vi "Tx_Create FIFO Association - Cyclic Labels - Disable Channels.vi"(8 "error in (no error)":errorcluster, 11 "Input Channel Data []":T3[](array[typedef]) {"Labels Settings"."Label Timestamp Channel Data Reference" format="%.0x"; "Labels Settings"."Label Disable/Trigger Channel Reference" format="%.0x"; "Labels Settings"."Word"."Param Setting"."Item Refs" format="%.0x"; "Labels Settings"."Word"."Param Setting"."Num Bits" min=1 max=32; "Labels Settings"."Word"."Param Setting"."Start Bit" min=8 max=31; "Labels Settings"."Label" format="%.0o"}) -> (0 "error out":errorcluster, 3 "Cyclic Labels - Disable Channels Map":T1[](array[typedef]) {"Channel Data Reference" format="%.0x"})   [LabVIEW 2016, in "Ballard Arinc-429 Engine.lvlib"]
doc: "This VI creates a static association between NI-VS FIFO Channel Index and Physical Channel, Label Index, of disable channel for a Tx Scheduled Label."
uses:
  Ballard Arinc-429 Engine.lvlib
  Shared/Controls and Global/RT HW Channel.ctl
  Shared/Controls and Global/RT Label Settings.ctl
  Shared/Controls and Global/Label.ctl
  Shared/Controls and Global/transferPeriod.ctl
  Shared/Controls and Global/RT Word Settings.ctl
  Shared/Controls and Global/RT Param Setting.ctl
  Shared/Controls and Global/Start Bit.ctl
  Shared/Controls and Global/Number of Bits.ctl
  <vilib>/NI Veristand/Custom Device API/Block Data Reference.ctl
  <vilib>/NI Veristand/Custom Device API/Data Reference.ctl
  <vilib>/NI Veristand/Custom Device API/Custom Device Item Ref.ctl
  Shared/Controls and Global/TransferType.ctl
  RT Controls/RT Tx Association.ctl
  <vilib>/NI VeriStand/Custom Device API/Custom Device API.lvlib
  Shared/Ballard Arinc-429 Shared.lvlib
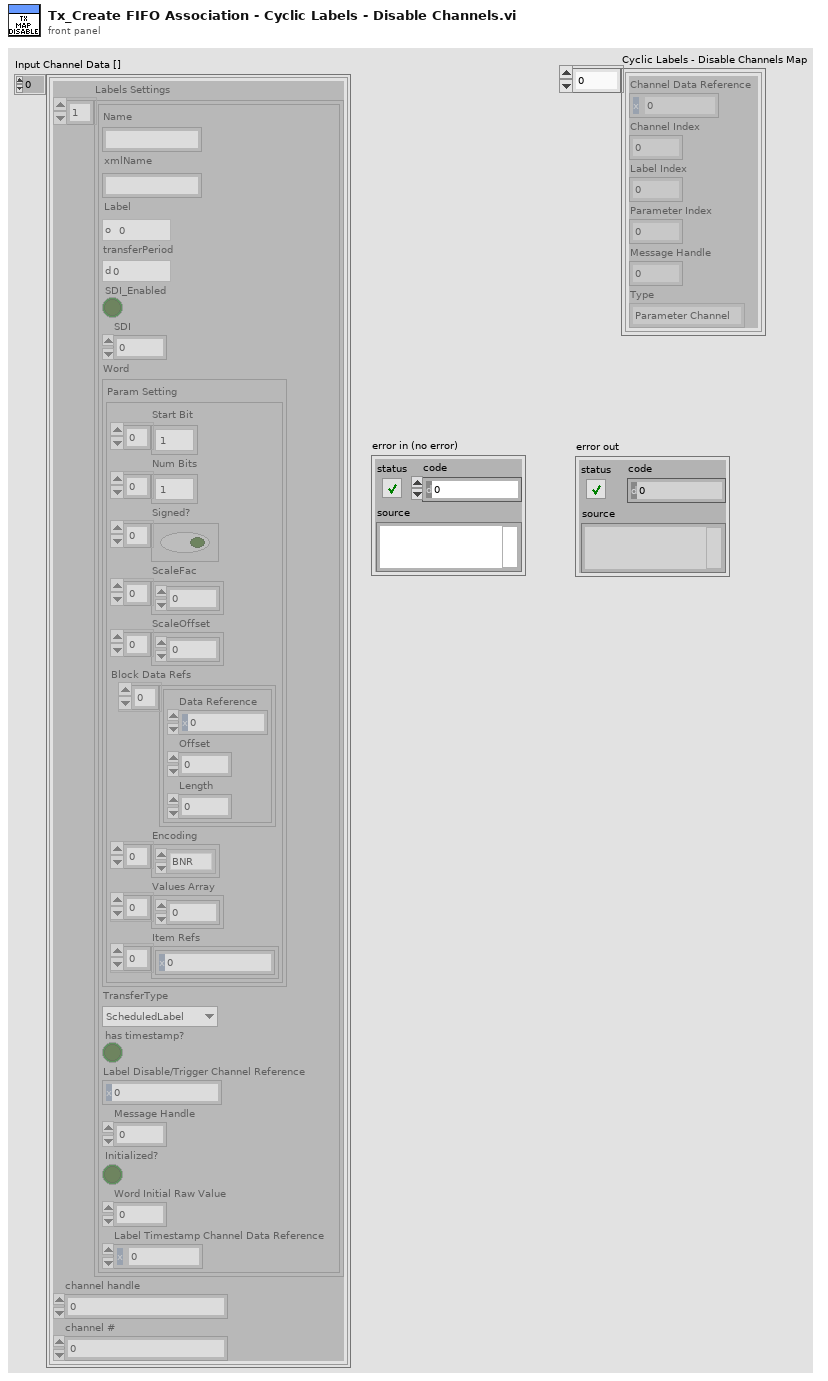
[diagram p1: front panel]
types:
  T1 = typedef "Ballard Arinc-429 Engine.lvlib/RT Tx Association.ctl" = cluster{"Channel Data Reference":T2, "Channel Index":i32, "Label Index":i32, "Parameter Index":i32, "Message Handle":u64, "Type":enum16{"Parameter Channel", "Disable/Trigger Channel"}}
  T2 = typedef "Custom Device API.lvlib/Data Reference.ctl" = i32
  T3 = typedef "Ballard Arinc-429 Shared.lvlib/RT HW Channel.ctl" = cluster{"Labels Settings":T4[], "channel handle":u64, "channel #":u16}
  T4 = typedef "Ballard Arinc-429 Shared.lvlib/RT Label Settings.ctl" = cluster{"Name":string, "xmlName":string, "Label":T5, "transferPeriod":T6, "SDI_Enabled":bool, "SDI":u8, "Word":T7, "TransferType":T13, "has timestamp?":bool, "Label Disable/Trigger Channel Reference":T12, "Message Handle":u64, "Initialized?":bool, "Word Initial Raw Value":u32, "Label Timestamp Channel Data Reference":T2}
  T5 = typedef "Ballard Arinc-429 Shared.lvlib/Label.ctl" = u8
  T6 = typedef "Ballard Arinc-429 Shared.lvlib/transferPeriod.ctl" = u32
  T7 = typedef "Ballard Arinc-429 Shared.lvlib/RT Word Settings.ctl" = cluster{"Param Setting":T8}
  T8 = typedef "Ballard Arinc-429 Shared.lvlib/RT Param Setting.ctl" = cluster{"Start Bit":T9[], "Num Bits":T10[], "Signed?":bool[], "ScaleFac":dbl[], "ScaleOffset":dbl[], "Block Data Refs":T11[], "Encoding":enum16{"BNR", "BCD", "Discrete"}[], "Values Array":dbl[], "Item Refs":T12[]}
  T9 = typedef "Ballard Arinc-429 Shared.lvlib/Start Bit.ctl" = i32
  T10 = typedef "Ballard Arinc-429 Shared.lvlib/Number of Bits.ctl" = i32
  T11 = typedef "Custom Device API.lvlib/Block Data Reference.ctl" = cluster{"Data Reference":T2, "Offset":u64, "Length":u64}
  T12 = typedef "Custom Device API.lvlib/Custom Device Item Ref.ctl" = u64
  T13 = typedef "Ballard Arinc-429 Shared.lvlib/TransferType.ctl" = enum16{"ScheduledLabel", "Acyclic", "Block", "Strobe"}
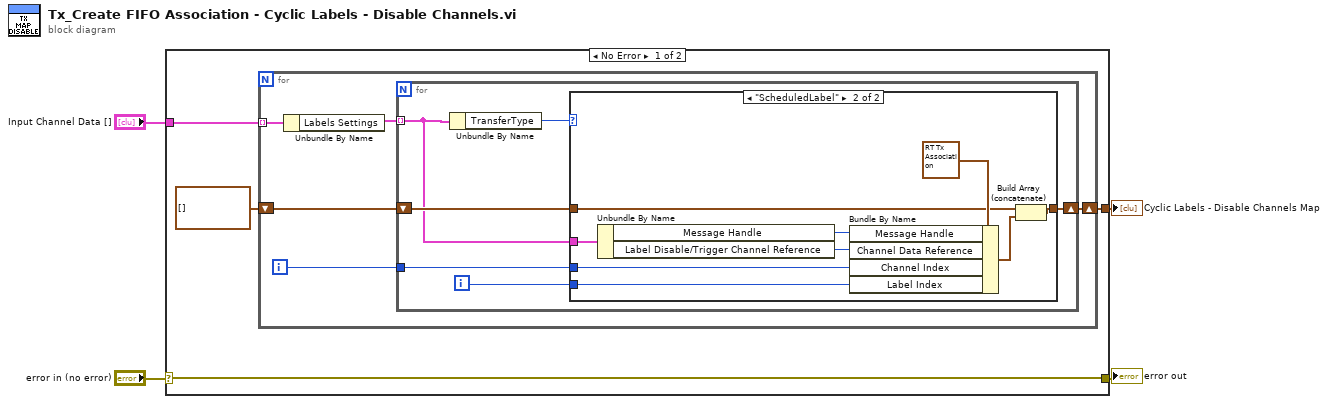
[diagram p0: block diagram]
diagram:
  n1 = case shown="No Error" "error in (no error)" {
    selector: "error in (no error)" -> [w6 w30]
    tunnel: [w6 w30] -> w3
    tunnel: "Input Channel Data []" -> [w8 _]
    tunnel: [w5 _] -> w1
    frame No Error {
      n2 = for {
        tunnel: w8 -> [w12] mode=indexing
        shift-right: [w9] -> w5
        shift-left: T1[] [] -> [w11]
        i -> [w10]
        n3 = Unbundle By Name(w12) -> ("Labels Settings"=w13:T4[])
        n4 = for {
          tunnel: w13 -> [w15] mode=indexing
          shift-right: [w16] -> w9
          shift-left: w11 -> [w18]
          tunnel: w10 -> [w19]
          i -> [w17]
          n5 = Unbundle By Name(w15) -> ("TransferType"=w14:T13)
          n6 = case shown="\"ScheduledLabel\"" w14 {
            tunnel: w19 -> [_ w28]
            tunnel: w18 -> [w20 w27]
            tunnel: w17 -> [_ w25]
            tunnel: [w20 w22] -> w16
            tunnel: w15 -> [_ w21]
            frame "Acyclic", Default {
            }
            frame "ScheduledLabel" {
              n7 = Unbundle By Name(w21) -> ("Message Handle"=w23:u64, "Label Disable/Trigger Channel Reference"=w24:T12)
              n8 = Bundle By Name(cluster=T1 {"Channel Data Reference"=0, "Channel Index"=0, "Label Index"=0, "Parameter Index"=-1, "Message Handle"=0, "Type"=enum."Disable/Trigger Channel"} ("Association"), "Message Handle"=w23, "Channel Data Reference"=w24, "Channel Index"=w28, "Label Index"=w25) -> (w26:T1)
              n9 = Build Array (concatenate)(w27, w26) -> (w22:T1[])
            }
          }
        }
      }
    }
    frame Error {
    }
  }
  "error out" <- w3
  "Cyclic Labels - Disable Channels Map" <- w1
